vi "SENS_CORR_EXT_PORT_FREQ.vi"(0 "VISA IN":refnum<visa-resource-name>, 1 "Port":i32, 2 "Frq. \"Use\" number":i32, 3 "Frq.":i32, 5 "error in":errorcluster, 7 "Channel":i32) -> (14 "VISA Out":refnum<visa-resource-name>, 19 "error out":errorcluster)   [LabVIEW 2018, in "PNA-X.lvlib"]
doc: "SENSe<cnum>:CORRection:EXTension:PORT<pnum>:FREQ<n> <value> \n(Read-Write) Sets and returns the frequency \"Use\" number (1|2) for the specified port number. \nLearn about Loss Compensation values. \nParameters \n<cnum> Any existing channel number. If unspecified, value is set to 1 \n<pnum> Port Number that will receive the freq/loss settings. If unspecified, value is set \nto 1. \n<n> Frequency \"Use\" number. Choose from 1 or 2. If unspecified, value is set to 1. \n<value> Frequency value. Choose a frequency within the frequency span of the PNA. \nExamples SENS:CORR:EXT:PORT1:FREQ1 10E9 \nsense2:correction:extension:port2:freq2:2E10 \nQuery Syntax SENSe<cnum>:CORRection:EXTension:PORT<pnum>:FREQ<n>? \nReturn Type Numeric \nDefault 1 GHz"
uses:
  PNA-X.lvlib
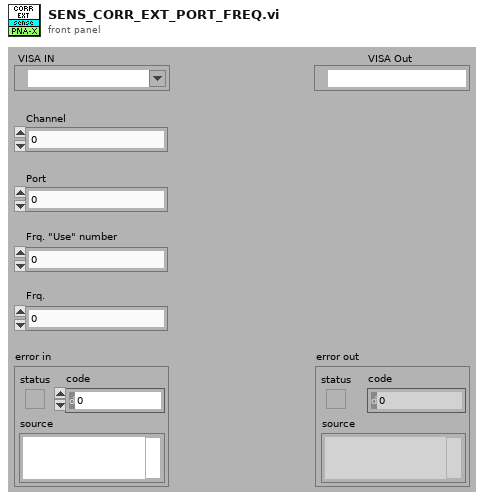
[diagram p1: front panel]
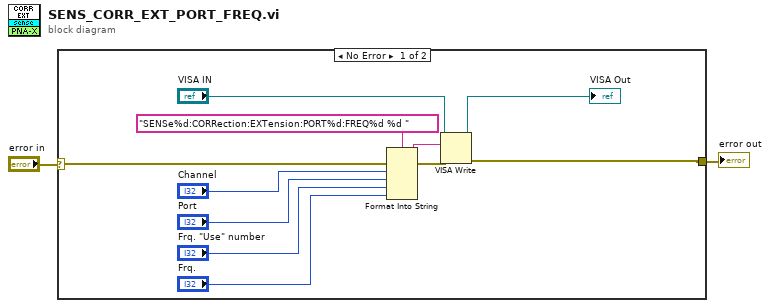
[diagram p0: block diagram]
diagram:
  n1 = case shown="No Error" "error in" {
    selector: "error in" -> [w13 w14]
    tunnel: [w8 w14] -> w1
    frame No Error {
      n2 = Format Into String(format string="SENSe%d:CORRection:EXTension:PORT%d:FREQ%d %d " ("Cmdline"), error in=w13, "Channel", "Port", "Frq. \"Use\" number", "Frq.") -> (resulting string=w11:string, error out=w12:errorcluster)  [unwired: 1 in]
      n3 = VISA Write(VISA resource name="VISA IN", write buffer=w11, error in (no error)=w12) -> (VISA resource name out=→"VISA Out":refnum<visa-resource-name>, error out=w8:errorcluster)  [unwired: 1 out]
    }
    frame Error {
    }
  }
  "error out" <- w1
